vi "Global Stop.vi"() -> ()   [LabVIEW 2014]
panel:
  out "Global Stop":bool
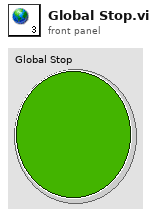
[diagram p1: front panel]
diagram:
